vi "HEWH Tdel Tin Average.vi"(7 "RTDout?":bool, 8 "error in (no error)":errorcluster, 11 "UEF Calculated Values Input":T1={"Calculated Values"={"Draw Cluster - Actual (Gal)"=[], "Mass of water All (lbm)"=[], "Density of hot water All (lbm/gal)"=[], "CpHW (BTU/(lbm °F))"=[], "rho 2 (lb/gal)"=0.0, "rho standby (lb/gal)"=0.0, "rho 24 (lb/gal)"=0.0, "Cp1 (BTU/(lb*F))"=0.0, "Cp2 (BTU/(lb*F))"=0.0, "Cp standby (BTU/(lb*F))"=0.0, "Cp 24 (BTU/(lb*F))"=0.0, "nu_r"=0.0, "Qstby (BTU)"=0.0, "Qhr (BTU/hr)"=0.0, "UA (BTU/(hr*F))"=0.0, "Q (BTU)"=0.0, "Qd (BTU)"=0.0, "Qda (BTU)"=0.0, "QHW67 (BTU)"=0.0, "UEF"=0.0, "Tdel1-Mean Outlet 1st Cluster(°F)"=0.0, "Tin1 - Mean Inlet 1st Cluster (°F)"=0.0, "Cp theoretical (BTU/(lbm °F))"=0.0, "M cluster mass removed (lb)"=0.0, "V1- Vol (Gal)"=0.0, "Test Data -Start to End"=[], "rho_nu (lb/gal)"=0.0, "Density of cold water All (lbm/gal)"=[], "CpUEF (BTU/(lb*F))"=0.0, "QHW (BTU)"=0.0, "QHWD (BTU)"=0.0, "Qdm (BTU)"=0.0, "FHD-After 1 Hour (String)"=[], "Vn"=0.0, "T*avg_del(n)"=0.0, "Max Location"=0, "T*min(n-1)"=0.0, "T*avg_del(n-1)"=0.0, "Full Credit?"=FALSE, "Temp Greater than T*min(n-1)"=FALSE, "Adjustment Factor"=0.0, "Draw Bonus Volume (gal)"=0.0}, "Sampled Data"={"Cold Water Draw Amounts-(Gal)"=[], "T del_all - Outlet Temps (°F)"=[], "T in_all - Inlet Temps (°F)"=[], "Qsu0 (BTU)"=14385.3, "Qsuf (BTU)"=15959.6, "Tau stby_1 (hr)"=8.4, "T suf(°F)"=125.0, "T su0(°F)"=126.1, "T tstby(°F)"=124.2, "T astby(°F)"=68.8, "T 24(°F)"=123.2, "Qr (BTU)"=7657.9, "T0 (°F)"=124.7, "Tmax1 (°F)"=124.8, "Qe (BTU)"=32770.2, "Qf (BTU)"=0.0, "Tastby2 (°F)"=68.9, "RTD Out Full Data\nSet (Each Draw)"=[], "RTD IN Full Data\nSet (Each Draw)"=[], "Tau stby2 (hr)"=23.406, "Hot Water Draw Amounts-(Gal)"=[], "Cold Flow Rate (GPM)"=[], "Hot Flow Rate (GPM)"=[], "Softw Elapsed Time\n Full Data Set (Each Draw)"=[], "Cold Gal Total Full\nData Set (Each Draw)"=[], "Total Hot Draw Amount (Gal) "=0.0, "Total Cold Draw Amount (Gal)"=0.0}, "Static Data"={"T-Wh Setpoint (°F)"=125.0, "T-Inlet Setpoint (°F)"=58.0, "T-Ambinet Nominal (°F)"=67.5, "V - Volume of Wh (True)"=46.0}, "Data Indexes"={"Test Start Index  (Full Index)"=0, "Header Length"=0, "Draw Index"=[], "Tmax1 Recovery Draw #"=0, "Start Watt Hours"=0.0, "Tsu0 Index"=0, "Tsf Index"=0, "Start Energy (BTU-Gas)"=0.0, "Usage Cluster"="", "T0 Index (Full Data Index)"=0, "Non-Draw Index"=[], "Tmax1 Index"=0, "Test End Index  (Full Index)"=0, "Heating Index"=[], "Heating Timestamp"=[], "Non-Draw Timestamp"=[], "Draw Index Timestamp"=[], "Tmax1 Timestamp"=0.0, "Tsu0 Timestamp"=0.0, "Tsf Timestamp"=0.0, "T0 Timestamp"=0.0, "Test End Timestamp"=0.0, "Test Start Timestamp"=0.0, "5 sec after Draw Timestamp"=[], "5 sec after Draw Index"=[], "Tmax1 Occurred During a Draw"=FALSE, "Usage Pattern (String)"="", "FHD Total Time (Sec)"=0.0}, "Raw Data"={"Elapsed Time Index"=0, "Software Elapsed Time Index"=0, "TC Tree Avg Index"=0, "Watt Hours (Wh) Index"=0, "Energy (BTU) Index"=0, "Totalized Flow Index"=0, "Flow Rate Index"=0, "Program Status Index"=0, "RTDin Index"=0, "RTDout Index"=0, "RTDamb Index"=0, "Test Data-Start to End DBL"=[], "Data Type"=enum."GEA Inlet Side Meter", "Heat Source Index"=0, "Hot Water Rate (GPM)"=0, "Hot Water Total (gal)"=0, "FHD-After 1 hour"=[]}, "Tolerance Check (T)=Pass"={"Flow Rate"=FALSE, "Totalized Flow"=FALSE, "Ambient Temp"=FALSE, "Ambient Humidity"=FALSE, "Inlet Temp"=FALSE, "Outlet Temp"=FALSE, "Valid Test"=FALSE, "Individual Totalized Flow"=FALSE, "Data Sheet Check"="", "Inlet Temperature"=[], "Tinlet Max"=[], "Tinlet Min"=[], "Flow Rate Max"=[], "Flow Rate Min"=[], "Amb Temp Max"=0.0, "Amb Temp Min"=0.0, "Toutlet Max"=0.0}, "Test Information"={"TR Number"="", "Lab ID"="", "Notes/Config"="", "Model Number"="", "Serial Number"="", "Lab Technician"="", "Engineer"="", "Type of Fuel"="", "Samp Received Date"="", "Samp Test Date"="", "Report Date"="", "Rate Input (kW or BTU/hr)"="", "Measured Input (kW or BTU/hr)"="", "Filename"=""}} {"Data Indexes"."5 sec after Draw Index" format="%#.2f"; "Data Indexes"."5 sec after Draw Timestamp" format="%#.2f"; "Data Indexes"."Test Start Timestamp" format="%.2f"; "Data Indexes"."Test End Timestamp" format="%.2f"; "Data Indexes"."T0 Timestamp" format="%.2f"; "Data Indexes"."Tsf Timestamp" format="%.2f"; "Data Indexes"."Tsu0 Timestamp" format="%.2f"; "Data Indexes"."Tmax1 Timestamp" format="%.2f"; "Data Indexes"."Draw Index Timestamp" format="%#.2f"; "Data Indexes"."Non-Draw Timestamp" format="%#.2f"; "Data Indexes"."Heating Timestamp" format="%#.2f"; "Data Indexes"."Start Energy (BTU-Gas)" format="%.6f"; "Data Indexes"."Start Watt Hours" format="%.6f"; "Static Data"."V - Volume of Wh (True)" format="%.5f"; "Static Data"."T-Ambinet Nominal (°F)" format="%.5f"; "Static Data"."T-Inlet Setpoint (°F)" format="%.5f"; "Static Data"."T-Wh Setpoint (°F)" format="%.5f"; "Sampled Data"."Tau stby2 (hr)" format="%.5f"; "Sampled Data"."Tastby2 (°F)" format="%.5f"; "Sampled Data"."Qf (BTU)" format="%.5f"; "Sampled Data"."Qe (BTU)" format="%.5f"; "Sampled Data"."Tmax1 (°F)" format="%.5f"; "Sampled Data"."T0 (°F)" format="%.5f"; "Sampled Data"."Qr (BTU)" format="%.5f"; "Sampled Data"."T 24(°F)" format="%.5f"; "Sampled Data"."T astby(°F)" format="%.5f"; "Sampled Data"."T tstby(°F)" format="%.5f"; "Sampled Data"."T su0(°F)" format="%.5f"; "Sampled Data"."T suf(°F)" format="%.5f"; "Sampled Data"."Tau stby_1 (hr)" format="%.5f"; "Sampled Data"."Qsuf (BTU)" format="%.5f"; "Sampled Data"."Qsu0 (BTU)" format="%.5f"; "Calculated Values"."Draw Bonus Volume (gal)" format="%.6f"; "Calculated Values"."Adjustment Factor" format="%.6f"; "Calculated Values"."T*avg_del(n-1)" format="%.6f"; "Calculated Values"."T*min(n-1)" format="%.6f"; "Calculated Values"."T*avg_del(n)" format="%.6f"; "Calculated Values"."Vn" format="%.6f"; "Calculated Values"."Qdm (BTU)" format="%.6f"; "Calculated Values"."QHWD (BTU)" format="%.6f"; "Calculated Values"."QHW (BTU)" format="%.6f"; "Calculated Values"."UEF" format="%.6f"; "Calculated Values"."QHW67 (BTU)" format="%.6f"; "Calculated Values"."Qda (BTU)" format="%.6f"; "Calculated Values"."Qd (BTU)" format="%.6f"; "Calculated Values"."Q (BTU)" format="%.6f"; "Calculated Values"."UA (BTU/(hr*F))" format="%.6f"; "Calculated Values"."Qhr (BTU/hr)" format="%.6f"; "Calculated Values"."Qstby (BTU)" format="%.6f"; "Calculated Values"."nu_r" format="%.6f"; "Calculated Values"."CpUEF (BTU/(lb*F))" format="%.6f"; "Calculated Values"."rho_nu (lb/gal)" format="%.6f"; "Calculated Values"."V1- Vol (Gal)" format="%.6f"; "Calculated Values"."M cluster mass removed (lb)" format="%.6f"; "Calculated Values"."Cp theoretical (BTU/(lbm °F))" format="%.6f"; "Calculated Values"."Tin1 - Mean Inlet 1st Cluster (°F)" format="%.6f"; "Calculated Values"."Tdel1-Mean Outlet 1st Cluster(°F)" format="%.6f"; "Calculated Values"."Cp 24 (BTU/(lb*F))" format="%.6f"; "Calculated Values"."Cp standby (BTU/(lb*F))" format="%.6f"; "Calculated Values"."Cp2 (BTU/(lb*F))" format="%.6f"; "Calculated Values"."Cp1 (BTU/(lb*F))" format="%.6f"; "Calculated Values"."rho 24 (lb/gal)" format="%.6f"; "Calculated Values"."rho standby (lb/gal)" format="%.6f"; "Calculated Values"."rho 2 (lb/gal)" format="%.6f"; "Calculated Values"."Density of cold water All (lbm/gal)" format="%#.3g"; "Calculated Values"."CpHW (BTU/(lbm °F))" format="%#.3g"; "Calculated Values"."Density of hot water All (lbm/gal)" format="%#.3g"; "Calculated Values"."Mass of water All (lbm)" format="%#.3f"}) -> (0 "error out":errorcluster, 1 "Draw Cluster - Actual (Gal)":dbl[](array[numeric]), 2 "V1":dbl, 3 "mean":dbl)   [LabVIEW 2019]
uses:
  Type Definitions/UEF Constants.ctl
  Type Definitions/HEWH Draw Stats.ctl
  Type Definitions/HEWH Usage Cluster.ctl
  Type Definitions/HEWH Meter Type.ctl
  <vilib>/Analysis/baseanly.llb/Mean (DBL).vi
  <vilib>/Analysis/NI_AALBase.lvlib
panel:
  out "Array":dbl[][](array[numeric])
  out "Tmax1 Timestamp":dbl
  out "Softw Elapsed Time\n Full Data Set (Each Draw)":dbl[][](array[numeric])
  out "Array 2":i32[][](array[numeric])
  # "FHR"
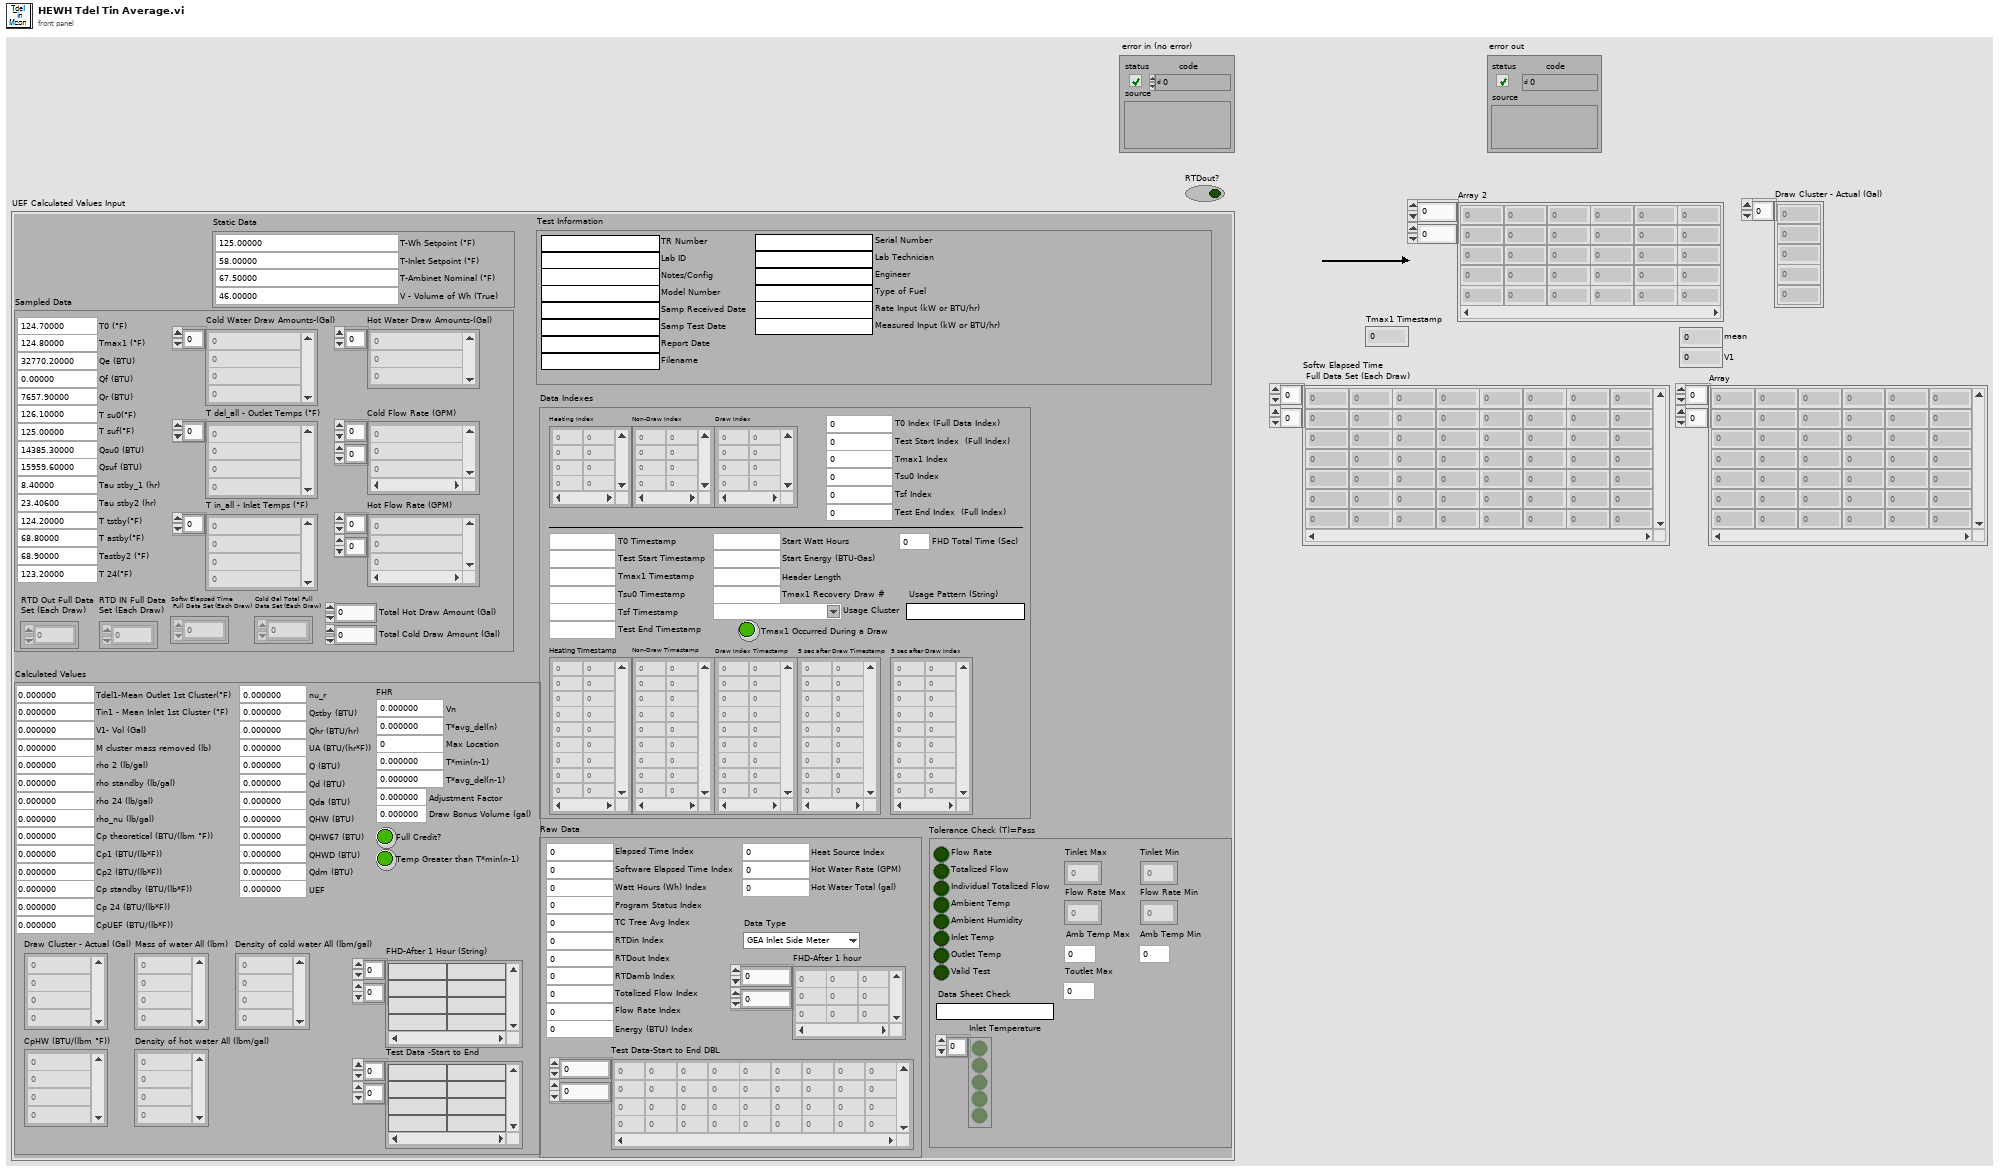
[diagram p1: front panel]
types:
  T1 = typedef "UEF Constants.ctl" = cluster{"Calculated Values":T2, "Sampled Data":cluster{"Cold Water Draw Amounts-(Gal)":dbl[], "T del_all - Outlet Temps (°F)":dbl[], "T in_all - Inlet Temps (°F)":dbl[], "Qsu0 (BTU)":dbl, "Qsuf (BTU)":dbl, "Tau stby_1 (hr)":dbl, "T suf(°F)":dbl, "T su0(°F)":dbl, "T tstby(°F)":dbl, "T astby(°F)":dbl, "T 24(°F)":dbl, "Qr (BTU)":dbl, "T0 (°F)":dbl, "Tmax1 (°F)":dbl, "Qe (BTU)":dbl, "Qf (BTU)":dbl, "Tastby2 (°F)":dbl, "RTD Out Full Data\nSet (Each Draw)":dbl[][], "RTD IN Full Data\nSet (Each Draw)":dbl[][], "Tau stby2 (hr)":dbl, "Hot Water Draw Amounts-(Gal)":dbl[], "Cold Flow Rate (GPM)":dbl[][], "Hot Flow Rate (GPM)":dbl[][], "Softw Elapsed Time\n Full Data Set (Each Draw)":dbl[][], "Cold Gal Total Full\nData Set (Each Draw)":dbl[][], "Total Hot Draw Amount (Gal) ":dbl, "Total Cold Draw Amount (Gal)":dbl}, "Static Data":cluster{"T-Wh Setpoint (°F)":dbl, "T-Inlet Setpoint (°F)":dbl, "T-Ambinet Nominal (°F)":dbl, "V - Volume of Wh (True)":dbl}, "Data Indexes":cluster{"Test Start Index  (Full Index)":i32, "Header Length":i32, "Draw Index":i32[][], "Tmax1 Recovery Draw #":i32, "Start Watt Hours":dbl, "Tsu0 Index":i32, "Tsf Index":i32, "Start Energy (BTU-Gas)":dbl, "Usage Cluster":T3, "T0 Index (Full Data Index)":i32, "Non-Draw Index":i32[][], "Tmax1 Index":i32, "Test End Index  (Full Index)":i32, "Heating Index":i32[][], "Heating Timestamp":dbl[][], "Non-Draw Timestamp":dbl[][], "Draw Index Timestamp":dbl[][], "Tmax1 Timestamp":dbl, "Tsu0 Timestamp":dbl, "Tsf Timestamp":dbl, "T0 Timestamp":dbl, "Test End Timestamp":dbl, "Test Start Timestamp":dbl, "5 sec after Draw Timestamp":dbl[][], "5 sec after Draw Index":dbl[][], "Tmax1 Occurred During a Draw":bool, "Usage Pattern (String)":string, "FHD Total Time (Sec)":dbl}, "Raw Data":cluster{"Elapsed Time Index":i32, "Software Elapsed Time Index":i32, "TC Tree Avg Index":i32, "Watt Hours (Wh) Index":i32, "Energy (BTU) Index":i32, "Totalized Flow Index":i32, "Flow Rate Index":i32, "Program Status Index":i32, "RTDin Index":i32, "RTDout Index":i32, "RTDamb Index":i32, "Test Data-Start to End DBL":dbl[][], "Data Type":T4, "Heat Source Index":i32, "Hot Water Rate (GPM)":i32, "Hot Water Total (gal)":i32, "FHD-After 1 hour":dbl[][]}, "Tolerance Check (T)=Pass":cluster{"Flow Rate":bool, "Totalized Flow":bool, "Ambient Temp":bool, "Ambient Humidity":bool, "Inlet Temp":bool, "Outlet Temp":bool, "Valid Test":bool, "Individual Totalized Flow":bool, "Data Sheet Check":string, "Inlet Temperature":bool[], "Tinlet Max":dbl[], "Tinlet Min":dbl[], "Flow Rate Max":dbl[], "Flow Rate Min":dbl[], "Amb Temp Max":dbl, "Amb Temp Min":dbl, "Toutlet Max":dbl}, "Test Information":cluster{"TR Number":string, "Lab ID":string, "Notes/Config":string, "Model Number":string, "Serial Number":string, "Lab Technician":string, "Engineer":string, "Type of Fuel":string, "Samp Received Date":string, "Samp Test Date":string, "Report Date":string, "Rate Input (kW or BTU/hr)":string, "Measured Input (kW or BTU/hr)":string, "Filename":string}}
  T2 = typedef "HEWH Draw Stats.ctl" = cluster{"Draw Cluster - Actual (Gal)":dbl[], "Mass of water All (lbm)":dbl[], "Density of hot water All (lbm/gal)":dbl[], "CpHW (BTU/(lbm °F))":dbl[], "rho 2 (lb/gal)":dbl, "rho standby (lb/gal)":dbl, "rho 24 (lb/gal)":dbl, "Cp1 (BTU/(lb*F))":dbl, "Cp2 (BTU/(lb*F))":dbl, "Cp standby (BTU/(lb*F))":dbl, "Cp 24 (BTU/(lb*F))":dbl, "nu_r":dbl, "Qstby (BTU)":dbl, "Qhr (BTU/hr)":dbl, "UA (BTU/(hr*F))":dbl, "Q (BTU)":dbl, "Qd (BTU)":dbl, "Qda (BTU)":dbl, "QHW67 (BTU)":dbl, "UEF":dbl, "Tdel1-Mean Outlet 1st Cluster(°F)":dbl, "Tin1 - Mean Inlet 1st Cluster (°F)":dbl, "Cp theoretical (BTU/(lbm °F))":dbl, "M cluster mass removed (lb)":dbl, "V1- Vol (Gal)":dbl, "Test Data -Start to End":string[][], "rho_nu (lb/gal)":dbl, "Density of cold water All (lbm/gal)":dbl[], "CpUEF (BTU/(lb*F))":dbl, "QHW (BTU)":dbl, "QHWD (BTU)":dbl, "Qdm (BTU)":dbl, "FHD-After 1 Hour (String)":string[][], "Vn":dbl, "T*avg_del(n)":dbl, "Max Location":i32, "T*min(n-1)":dbl, "T*avg_del(n-1)":dbl, "Full Credit?":bool, "Temp Greater than T*min(n-1)":bool, "Adjustment Factor":dbl, "Draw Bonus Volume (gal)":dbl}
  T3 = typedef "HEWH Usage Cluster.ctl" = string
  T4 = typedef "HEWH Meter Type.ctl" = enum16{"GEA Inlet Side Meter", "GEA Outlet Side Meter", "CSA Inlet Side Meter"}
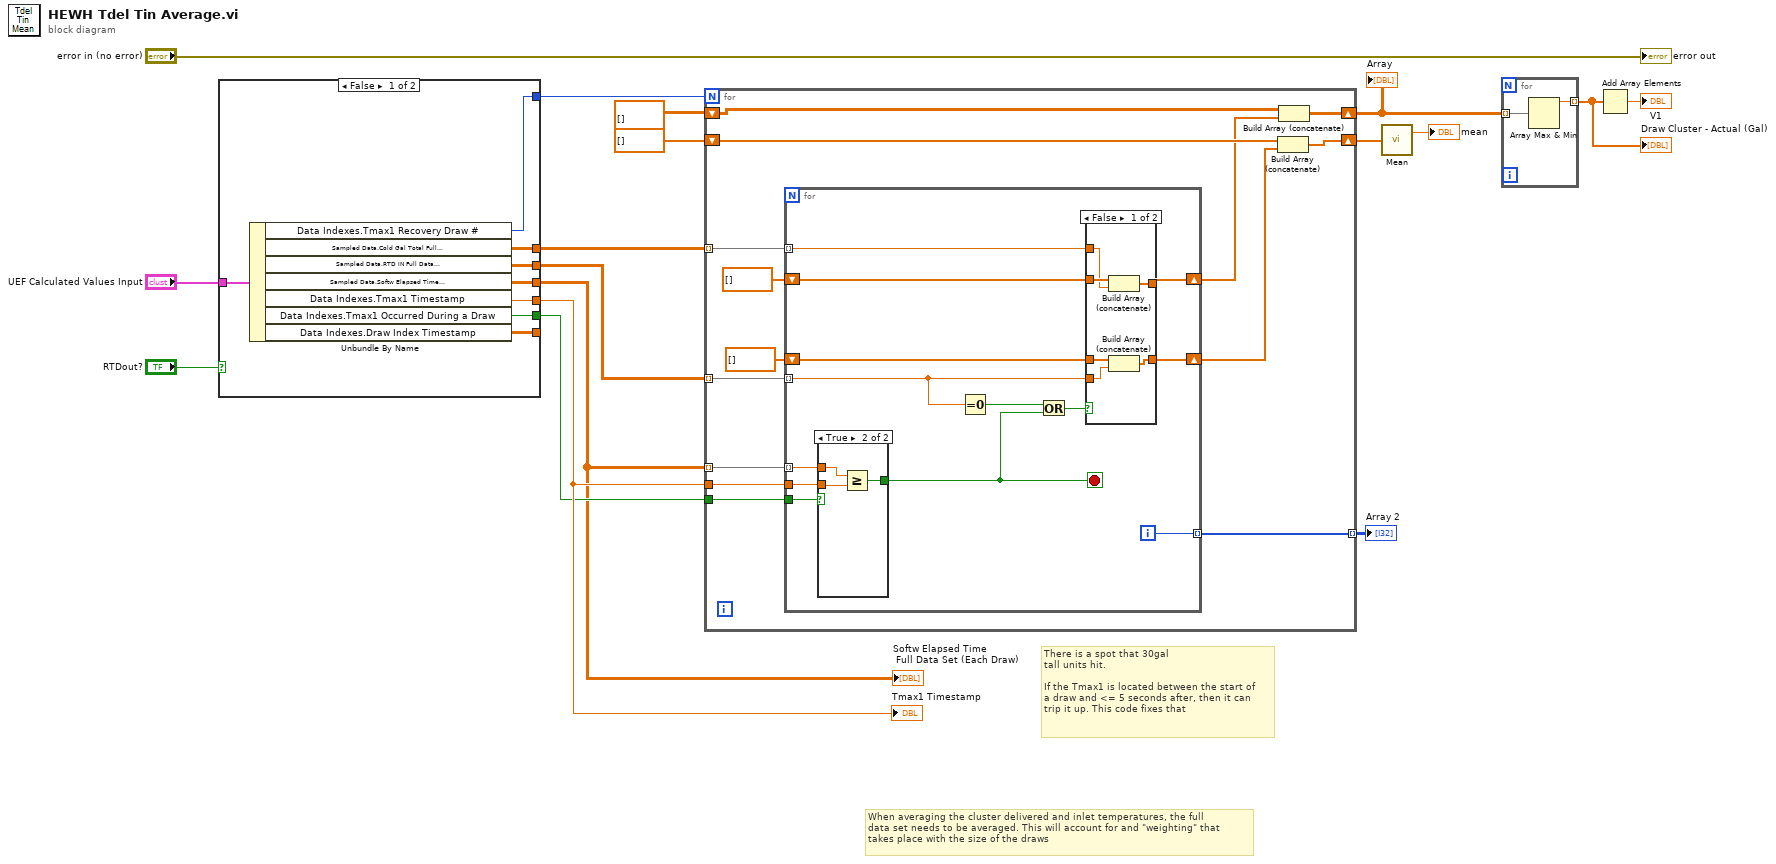
[diagram p0: block diagram]
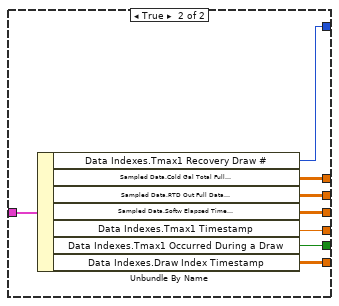
[diagram p2: hidden frame]
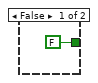
[diagram p3: hidden frame]
diagram:
  # "There is a spot that 30gal\ntall units hit.\n\nIf the Tmax1 is located between the start of \na draw and <= 5 seconds after, then it can \ntrip it up. This code fixes that"
  # "When averaging the cluster delivered and inlet temperatures, the full \ndata set needs to be averaged. This will account for and \"weighting\" that \ntakes place with the size of the draws"
  n1 = case shown="False" "RTDout?" {
    tunnel: "UEF Calculated Values Input" -> [w25 w33]
    tunnel: [w24 w32] -> w11
    tunnel: [w23 w31] -> w1
    tunnel: [w22 w30] -> w2
    tunnel: [w21 w29] -> w10
    tunnel: [w20 w28] -> w9
    tunnel: [w19 w27] -> w7
    tunnel: [w18 w26] -> _
    frame False {
      n2 = Unbundle By Name(w25) -> ("Data Indexes.Tmax1 Recovery Draw #"=w24:i32, "Sampled Data.Cold Gal Total Full\nData Set (Each Draw)"=w19:dbl[][], "Sampled Data.RTD IN Full Data\nSet (Each Draw)"=w23:dbl[][], "Sampled Data.Softw Elapsed Time\n Full Data Set (Each Draw)"=w22:dbl[][], "Data Indexes.Tmax1 Timestamp"=w21:dbl, "Data Indexes.Tmax1 Occurred During a Draw"=w20:bool, "Data Indexes.Draw Index Timestamp"=w18:dbl[][])
    }
    frame True {
      n3 = Unbundle By Name(w33) -> ("Data Indexes.Tmax1 Recovery Draw #"=w32:i32, "Sampled Data.Cold Gal Total Full\nData Set (Each Draw)"=w27:dbl[][], "Sampled Data.RTD Out Full Data\nSet (Each Draw)"=w31:dbl[][], "Sampled Data.Softw Elapsed Time\n Full Data Set (Each Draw)"=w30:dbl[][], "Data Indexes.Tmax1 Timestamp"=w29:dbl, "Data Indexes.Tmax1 Occurred During a Draw"=w28:bool, "Data Indexes.Draw Index Timestamp"=w26:dbl[][])
    }
  }
  "Softw Elapsed Time\n Full Data Set (Each Draw)" <- w2
  "Tmax1 Timestamp" <- w10
  n4 = for {
    N: w11 -> [_]
    tunnel: w1 -> [w45] mode=indexing
    shift-right: [w46] -> w16
    shift-left: dbl[] [] -> [w47]
    tunnel: w2 -> [w42] mode=indexing
    tunnel: w9 -> [w41]
    tunnel: w10 -> [w40]
    tunnel: [w39] -> w13 mode=indexing
    tunnel: w7 -> [w38] mode=indexing
    shift-right: [w34] -> w5
    shift-left: dbl[][] [] -> [w36]
    n5 = for {
      tunnel: w45 -> [w58] mode=indexing
      shift-right: [w59] -> w43
      shift-left: dbl[] [] -> [w60]
      tunnel: w42 -> [w55] mode=indexing
      tunnel: w41 -> [w57]
      tunnel: w40 -> [w56]
      tunnel: [w54] -> w39 mode=indexing
      tunnel: w38 -> [w52] mode=indexing
      shift-right: [w51] -> w35
      shift-left: dbl[] [] -> [w53]
      i -> [w54]
      stop <- w49 stop-if-true
      n6 = case shown="True" w57 {
        tunnel: w56 -> [_ w63]
        tunnel: w55 -> [_ w64]
        tunnel: [FALSE w62] -> w49
        frame False {
        }
        frame True {
          n7 = Greater Or Equal?(x=w64, y=w63) -> (x >= y?=w62:bool)
        }
      }
      n8 = Equal To 0?(x=w58) -> (x = 0?=w50:bool)
      n9 = Or(x=w50, y=w49) -> (x .or. y?=w48:bool)
      n10 = case shown="False" w48 {
        tunnel: w60 -> [w70 w72]
        tunnel: [w69 w72] -> w59
        tunnel: w58 -> [w68 _]
        tunnel: w53 -> [w67 w71]
        tunnel: w52 -> [w66 _]
        tunnel: [w65 w71] -> w51
        frame False {
          n11 = Build Array (concatenate)(w67, w66) -> (w65:dbl[])
          n12 = Build Array (concatenate)(w70, w68) -> (w69:dbl[])
        }
        frame True {
        }
      }
    }
    n13 = Build Array (concatenate)(w47, w43) -> (w46:dbl[])
    n14 = Build Array (concatenate)(w36, w35) -> (w34:dbl[][])
  }
  "Array 2" <- w13
  "Array" <- w5
  n15 = call-poly <vilib>:"Mean.vi"("X"=w16) -> ("mean"=→"mean":dbl)  [unwired: 1 out]
  n16 = for {
    tunnel: w5 -> [w74] mode=indexing
    tunnel: [w73] -> w4 mode=indexing
    n17 = Array Max & Min(array=w74) -> (max value=w73:dbl)  [unwired: 3 out]
  }
  "Draw Cluster - Actual (Gal)" <- w4
  n18 = Add Array Elements(numeric array=w4) -> (sum=→"V1":dbl)
  "error out" <- "error in (no error)"
